vi "http option action.vi"(11 "application request in":T1) -> (3 "application request out":T4)   [LabVIEW 2016, in "http responder.lvclass"]
uses:
  http responder.lvclass
  HTTP server/http response.ctl
  HTTP server/http response packet type.ctl
  HTTP headers/http header data.ctl
  HTTP server/http request.ctl
  HTTP server/http method.ctl
  HTTP server/Basic HTTP server.lvclass
  HTTP headers/http headers.lvlib
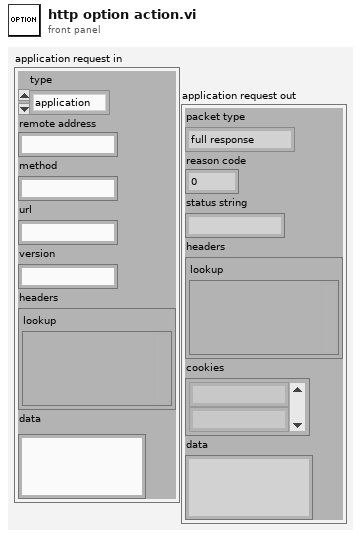
[diagram p1: front panel]
types:
  T1 = typedef "Basic HTTP server.lvclass/http request.ctl" = cluster{"type":T2, "remote address":string, "method":string, "url":string, "version":string, "headers":T3, "data":string}
  T2 = typedef "Basic HTTP server.lvclass/http method.ctl" = enum16{"application", "error", "upgrade", "expect"}
  T3 = typedef "http headers.lvlib/http header data.ctl" = cluster{"lookup":variant}
  T4 = typedef "Basic HTTP server.lvclass/http response.ctl" = cluster{"packet type":T5, "reason code":u16, "status string":string, "headers":T3, "cookies":string[], "data":string}
  T5 = typedef "Basic HTTP server.lvclass/http response packet type.ctl" = enum16{"full response", "header only", "data only", "last data", "raw output"}
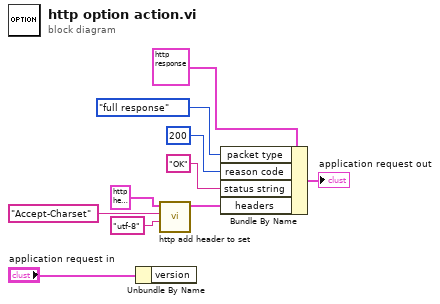
[diagram p0: block diagram]
diagram:
  n1 = Unbundle By Name("application request in") -> ()  [unwired: 1 out]
  n2 = call "http add header to set.vi"("header field data"="utf-8" ("name"), "header field name"="Accept-Charset" ("name"), "headers in"=T3 {"lookup"=variant}) -> ("headers out"=w1:T3)  [unwired: 8 in]
  n3 = Bundle By Name(cluster=T4 {"packet type"=enum."full response", "reason code"=0, "status string"="", "headers"={"lookup"=variant}, "cookies"=[], "data"=""} ("application request"), "packet type"=http_response_packet_type."full response", "reason code"=u16 200, "status string"="OK", "headers"=w1) -> (→"application request out":T4)
